vi "AB_Log_Enable_Logging.vi"(8 "error in (no error)":errorcluster, 11 "read INI":bool) -> (0 "error out":errorcluster, 1 "use LLB for app":bool, 2 "save twice?":bool, 3 "log?":bool, 4 "keep internal.llb":bool, 5 "check VI state during copy":bool, 6 "save mode":T1=enum."save", 7 "sdist_exclude_edittime":bool)   [LabVIEW 2020]
uses:
  <vilib>/AppBuilder/logging/AB_Log_Save_Action.ctl
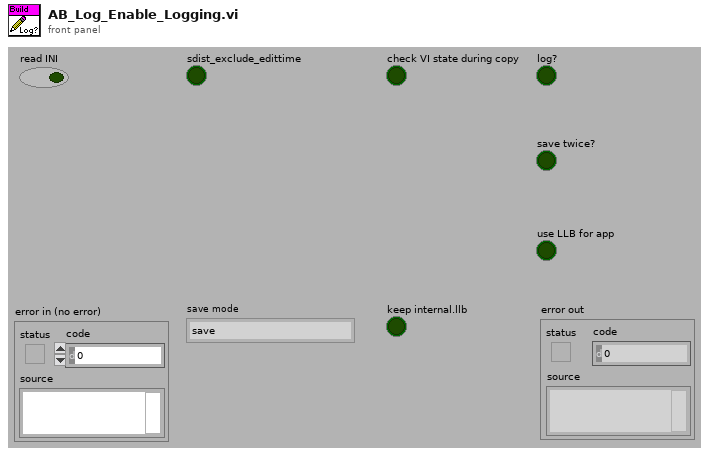
[diagram p1: front panel]
types:
  T1 = typedef "AB_Log_Save_Action.ctl" = enum32{"consolidated save with types", "consolidated save", "save"}
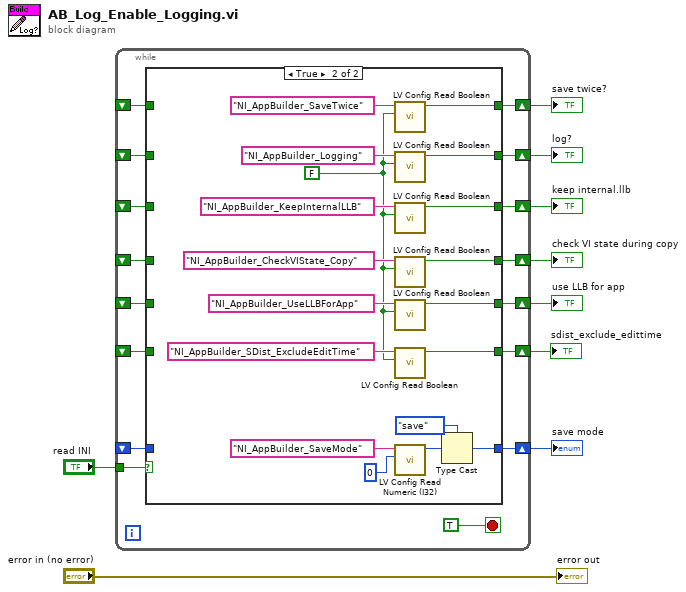
[diagram p0: block diagram]
diagram:
  n1 = while {
    shift-right: [w24] -> w7
    shift-left: _ -> [w22]
    tunnel: "read INI" -> [w23]
    shift-right: [w20] -> w6
    shift-left: _ -> [w21]
    shift-right: [w19] -> w5
    shift-left: _ -> [w18]
    shift-right: [w17] -> w4
    shift-left: _ -> [w16]
    shift-right: [w15] -> w3
    shift-left: _ -> [w14]
    shift-right: [w13] -> w2
    shift-left: _ -> [w12]
    shift-right: [w11] -> w1
    shift-left: _ -> [w10]
    stop <- TRUE stop-if-true
    n2 = case shown="True" w23 {
      tunnel: [w32 w50] -> w24
      tunnel: w22 -> [w32 _]
      tunnel: [w31 w48] -> w20
      tunnel: w21 -> [w31 _]
      tunnel: [w30 w45] -> w19
      tunnel: w18 -> [w30 _]
      tunnel: [w29 w43] -> w17
      tunnel: w16 -> [w29 _]
      tunnel: [w28 w42] -> w15
      tunnel: w14 -> [w28 _]
      tunnel: [w27 w36] -> w13
      tunnel: w12 -> [w27 _]
      tunnel: [w26 w34] -> w11
      tunnel: w10 -> [w26 _]
      frame False {
      }
      frame True {
        w33 = FALSE ("default value")
        n3 = call <resource>:"LV Config Read Boolean.vi"("default value"=w33, "key"="NI_AppBuilder_SaveTwice") -> ("value"=w45:bool)  [unwired: 1 in, 4 out]
        n4 = call <resource>:"LV Config Read Boolean.vi"("default value"=w33, "key"="NI_AppBuilder_Logging") -> ("value"=w50:bool)  [unwired: 1 in, 4 out]
        n5 = call <resource>:"LV Config Read Boolean.vi"("default value"=w33, "key"="NI_AppBuilder_KeepInternalLLB") -> ("value"=w48:bool)  [unwired: 1 in, 4 out]
        n6 = call <resource>:"LV Config Read Boolean.vi"("default value"=w33, "key"="NI_AppBuilder_CheckVIState_Copy") -> ("value"=w43:bool)  [unwired: 1 in, 4 out]
        n7 = call <resource>:"LV Config Read Boolean.vi"("default value"=w33, "key"="NI_AppBuilder_UseLLBForApp") -> ("value"=w42:bool)  [unwired: 1 in, 4 out]
        n8 = call <resource>:"LV Config Read Boolean.vi"("default value"=w33, "key"="NI_AppBuilder_SDist_ExcludeEditTime") -> ("value"=w34:bool)  [unwired: 1 in, 4 out]
        n9 = call <resource>:"LV Config Read Numeric (I32).vi"("default value"=0, "key"="NI_AppBuilder_SaveMode") -> ("value"=w37:i32)  [unwired: 3 in, 2 out]
        n10 = Type Cast(type=AB_Log_Save_Action."save" ("fileAction"), x=w37) -> (*(type *) &x=w36:T1)
      }
    }
  }
  "log?" <- w7
  "keep internal.llb" <- w6
  "save twice?" <- w5
  "check VI state during copy" <- w4
  "use LLB for app" <- w3
  "save mode" <- w2
  "sdist_exclude_edittime" <- w1
  "error out" <- "error in (no error)"
